vi "Compute Pseudo-Phase Lifetime Plot.vi"(8 "Error In":errorcluster, 9 "Compute Delta Tau":bool, 10 "Phasor Parameters":T1={"Display Parameters"={"# Points"=0, "Ramp Type"=enum."Linear", "Type of Series"=enum."1-Exp Decays", "Min tau"=0.0, "Max tau"=0.0, "Include 0"=FALSE, "Include Infinity"=FALSE}, "Phasor Parameters"={"Harmonic frequency"=0.0, "Use f* = 1/D Frequency"=FALSE, "Calibrated Phasor"=FALSE, "Calibration Lifetime"=1e-09, "Phasor Calculation"=enum."Direct Sum", "SEPL Type"=enum."UC", "# Gates"=1.0, "Square Gate Width"=1e-09, "Show Ticks"=FALSE}, "Decay & IRF Parameters"={"Lifetime"=0.0, "IRF Offset"=0.0, "Laser Period"=0.0, "Normalized Decays"=FALSE, "IRF Model"=enum."Dirac", "IRF Parameter 1"=0.0}, "Gate Parameters"={"First Gate Start"=0.0, "Use Gate Center"=FALSE, "Gate Width"=0.0, "Gate Step"=0.0, "# Gates"=0.0, "Gate Type"=enum."Square", "Edge Width"=0.0, "Top Slope"=0.0, "Reversed Sawtooth?"=FALSE, "Analytical Computation"=FALSE, "Tolerance"=1.0, "Integration"=enum."Item 0", "# Steps"=1.0, "Type of User-defined Function"=enum."Gate"}, "Detector Parameters"={"Frames/Image"=0, "Gates/Frame"=0, "Bits/Frame"=0, "Multiplicity"=0, "Incident Signal"=0.0}} {"Detector Parameters"."Frames/Image" min=1; "Detector Parameters"."Multiplicity" min=0; "Detector Parameters"."Bits/Frame" min=1; "Detector Parameters"."Gates/Frame" min=1; "Gate Parameters"."# Steps" min=0.0; "Gate Parameters"."Tolerance" min=0.0; "Gate Parameters"."Top Slope" min=0.0; "Gate Parameters"."Edge Width" min=0.0; "Gate Parameters"."Gate Step" min=0.0; "Gate Parameters"."# Gates" min=0.0 step=1.0; "Gate Parameters"."Gate Width" min=0.0; "Decay & IRF Parameters"."Lifetime" min=0.0; "Decay & IRF Parameters"."Laser Period" min=0.0; "Phasor Parameters"."Square Gate Width" min=0.0; "Phasor Parameters"."# Gates" min=0.0; "Phasor Parameters"."Calibration Lifetime" min=0.0; "Phasor Parameters"."Harmonic frequency" min=0.0; "Display Parameters"."Min tau" min=0.0; "Display Parameters"."Max tau" min=0.0; "Display Parameters"."# Points" min=1 step=1}, 11 "P-tau_ph(tau) Graph Refnum":refnum<vi>) -> (0 "Error Out":errorcluster)   [LabVIEW 2019]
uses:
  Pseudo Phasor Parameters.ctl
  Phasor Explorer Display Parameters.ctl
  Type of Series.ctl
  Phasor Explorer Phasor Parameters.ctl
  Phasor Calculation Type.ctl
  Phasor Type.ctl
  Phasor Explorer Decay Parameters.ctl
  IRF Model.ctl
  Phasor Explorer Gate Parameters.ctl
  Gate Type.ctl
  Phasor Explorer Detector Parameters.ctl
  Phasor UC_N[W] Parameters.ctl
  <vilib>/Utility/error.llb/Error Cluster From Error Code.vi
  SEPXP Globals.vi
  <vilib>/ErrorRing/Error Ring.xnode
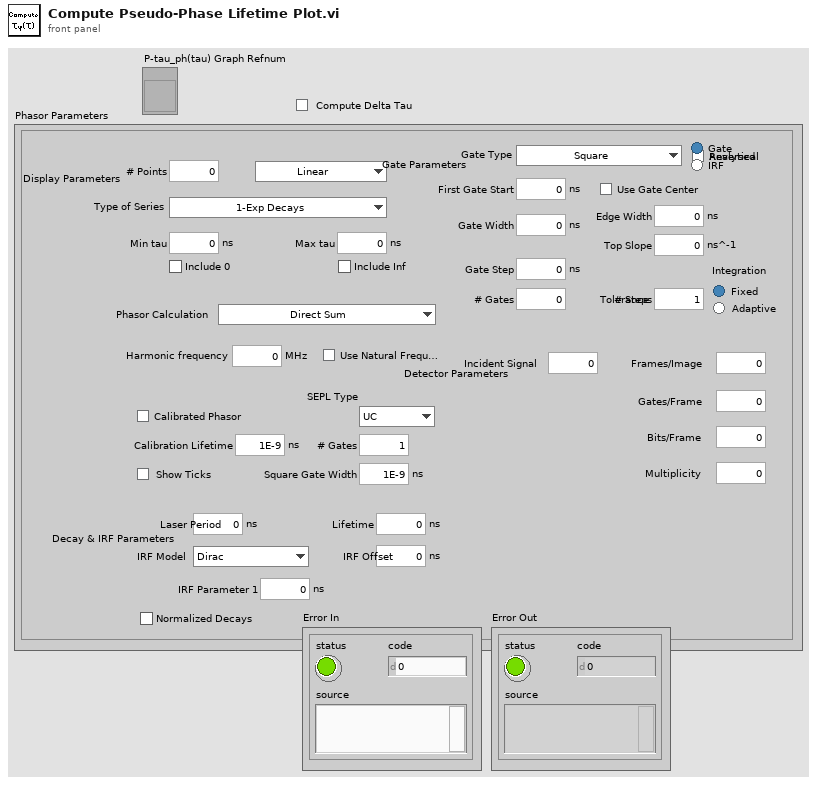
[diagram p1: front panel]
types:
  T1 = typedef "Pseudo Phasor Parameters.ctl" = cluster{"Display Parameters":T2, "Phasor Parameters":T4, "Decay & IRF Parameters":T7, "Gate Parameters":T9, "Detector Parameters":T11}
  T2 = typedef "Phasor Explorer Display Parameters.ctl" = cluster{"# Points":i32, "Ramp Type":enum16{"Linear", "Logarithmic"}, "Type of Series":T3, "Min tau":dbl[unit], "Max tau":dbl[unit], "Include 0":bool, "Include Infinity":bool}
  T3 = typedef "Type of Series.ctl" = enum16{"1-Exp Decays", "Linear Combination of 1-Exp"}
  T4 = typedef "Phasor Explorer Phasor Parameters.ctl" = cluster{"Harmonic frequency":dbl[unit], "Use f* = 1/D Frequency":bool, "Calibrated Phasor":bool, "Calibration Lifetime":dbl[unit], "Phasor Calculation":T5, "SEPL Type":T6, "# Gates":dbl, "Square Gate Width":dbl[unit], "Show Ticks":bool}
  T5 = typedef "Phasor Calculation Type.ctl" = enum16{"Direct Sum", "Analytical Formula"}
  T6 = typedef "Phasor Type.ctl" = enum16{"UC", "L_N", "L_N[W]"}
  T7 = typedef "Phasor Explorer Decay Parameters.ctl" = cluster{"Lifetime":dbl[unit], "IRF Offset":dbl[unit], "Laser Period":dbl[unit], "Normalized Decays":bool, "IRF Model":T8, "IRF Parameter 1":dbl[unit]}
  T8 = typedef "IRF Model.ctl" = enum16{"Dirac", "Exponential"}
  T9 = typedef "Phasor Explorer Gate Parameters.ctl" = cluster{"First Gate Start":dbl[unit], "Use Gate Center":bool, "Gate Width":dbl[unit], "Gate Step":dbl[unit], "# Gates":dbl, "Gate Type":T10, "Edge Width":dbl[unit], "Top Slope":dbl[unit], "Reversed Sawtooth?":bool, "Analytical Computation":bool, "Tolerance":dbl, "Integration":enum32{"Item 0", "Item 1"}, "# Steps":dbl, "Type of User-defined Function":enum32{"Gate", "IRF"}}
  T10 = typedef "Gate Type.ctl" = enum16{"Square", "Finite Edge Square", "Finite Edge, Tilted Top Square", "Triangle", "Sawtooth", "User-defined"}
  T11 = typedef "Phasor Explorer Detector Parameters.ctl" = cluster{"Frames/Image":i32, "Gates/Frame":i32, "Bits/Frame":i32, "Multiplicity":i32, "Incident Signal":dbl}
  T12 = typedef "Phasor UC_N[W] Parameters.ctl" = cluster{"Laser Period":dbl[unit], "Gate Width":dbl[unit], "Gate Step":dbl[unit], "Harmonic frequency":dbl[unit], "IRF offset":dbl[unit], "# Gates":dbl}
  T13 = typedef "Gate Definitions.ctl" = cluster{"First Gate: t1":ext, "Gate Width: W":ext, "Gate Step: d":ext, "# Gates: G":ext, "Use Gate Center":bool, "Frames/Image: F":i32, "Gates/Frame: L":i32, "Bits/Frame: q":i32, "Multiplicity: p":i32, "Gate Type":T10, "Gate Edge s":ext, "Gate Top Slope":ext, "Reversed Sawtooth?":bool, "Computation":bool, "User-defined Gate":T14, "Tolerance":ext, "Integration":enum32{"Item 0", "Item 1"}, "# Steps":ext, "Type of User-defined Function":enum32{"Gate", "IRF"}}
  T14 = typedef "XY Plot Data.ctl" = cluster{"X Array":dbl[], "Y Array":dbl[]}
  T15 = typedef "Decay Definiton.ctl" = cluster{"offset: t0":ext, "period: T":ext, "lifetime: tau":ext, "Incident Signal: I":ext, "Normalized Decays":bool, "IRF Model":T8, "IRF Parameter 1":ext}
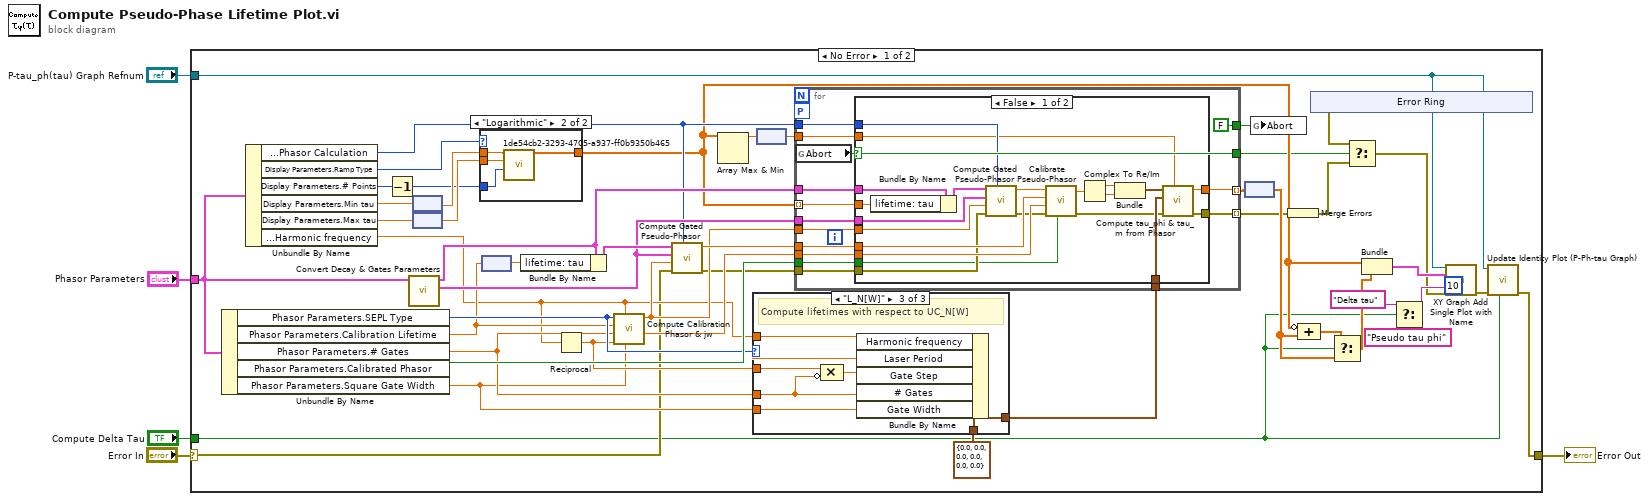
[diagram p0: block diagram]
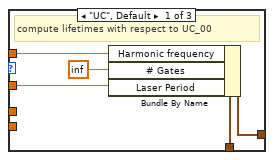
[diagram p2: hidden frame]
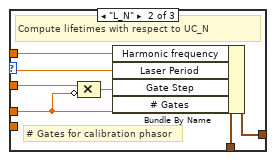
[diagram p3: hidden frame]
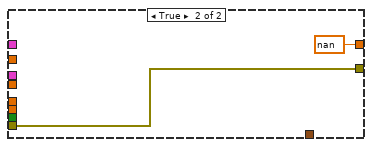
[diagram p4: hidden frame]
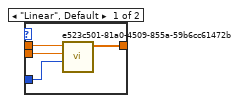
[diagram p5: hidden frame]
diagram:
  n1 = case shown="No Error" "Error In" {
    selector: "Error In" -> [w8 w122]
    tunnel: "Phasor Parameters" -> [w22 _]
    tunnel: "P-tau_ph(tau) Graph Refnum" -> [w41 _]
    tunnel: [w39 w122] -> w2
    tunnel: "Compute Delta Tau" -> [w6 _]
    frame No Error {
      (unwired) 10 ("Max Legend Size (8)")
      n2 = Unbundle By Name(w22) -> ("Phasor Parameters.SEPL Type"=w23:T6, "Phasor Parameters.Calibration Lifetime"=w18:dbl[unit], "Phasor Parameters.# Gates"=w19:dbl, "Phasor Parameters.Calibrated Phasor"=w36:bool, "Phasor Parameters.Square Gate Width"=w11:dbl[unit])
      n3 = Unbundle By Name(w22) -> ("Phasor Parameters.Phasor Calculation"=w35:T5, "Display Parameters.Ramp Type"=w44:enum16{"Linear", "Logarithmic"}, "Display Parameters.# Points"=w43:i32, "Display Parameters.Min tau"=w52:dbl[unit], "Display Parameters.Max tau"=w53:dbl[unit], "Phasor Parameters.Harmonic frequency"=w17:dbl[unit])
      n4 = Decrement(x=w43) -> (x-1=w42:i32)
      n5 = call "Convert Decay & Gates Parameters.vi"("Phasor Parameters"=w22) -> ("Gates Definitions"=w37:T13, "Decay Definition"=w38:T15)  [unwired: 9 in]
      n6 = node(w52) -> (w46:dbl)
      n7 = node(w53) -> (w47:dbl)
      n8 = case shown="\"Logarithmic\"" w44 {
        tunnel: w47 -> [w117 w119]
        tunnel: w46 -> [w116 w120]
        tunnel: [w115 w118] -> w26
        tunnel: w42 -> [w114 w121]
        frame "Linear", Default {
          n9 = call "e523c501-81a0-4509-855a-59b6cc61472b.vi"("# Steps (1)"=w114, "End (1)"=w117, "Start (0)"=w116) -> ("Ramp"=w115:dbl[])  [unwired: 7 in, 1 out]
        }
        frame "Logarithmic" {
          n10 = call "1de54cb2-3293-4705-a937-ff0b9350b465.vi"("# Steps (1)"=w121, "End (1)"=w119, "Start (1)"=w120) -> ("Ramp"=w118:dbl[])  [unwired: 7 in, 1 out]
        }
      }
      n11 = node(w18) -> (w49:dbl)
      n12 = Bundle By Name(cluster=w38, "lifetime: tau"=w49) -> (w50:T15)
      n13 = Reciprocal(x=w17) -> (1/x=w16:dbl[unit])
      n14 = call "Compute Calibration Phasor & jw.vi"("Gate Width"=w11, "Harmonic frequency"=w17, "Laser Period"=w16, "# Gates"=w19, "Calibration Lifetime"=w18, "Calibration Phasor Type"=w23) -> ("z (tau_cal)"=w27:cdb, "i 2 pi f (GHz)"=w28:cdb)  [unwired: 4 in]
      n15 = call "Compute Gated Pseudo-Phasor.vi"("Phasor Calculation Type"=w35, "Error In"=w8, "j 2 pi f"=w28, "Gates Definitions"=w37, "Decay Definition"=w50) -> ("Error Out"=w10:errorcluster, "phasor"=w48:cxt)  [unwired: 4 in, 1 out]
      n16 = Array Max & Min(array=w26) -> (max value=w25:dbl)  [unwired: 3 out]
      n17 = case shown="\"L_N[W]\"" w23 {
        tunnel: [w62 w68 w75] -> w21
        tunnel: T12 {"Laser Period"=0.0, "Gate Width"=0.0, "Gate Step"=0.0, "Harmonic frequency"=0.0, "IRF offset"=0.0, "# Gates"=0.0} ("Phasor UCN[W] Parameters") -> [w60 w67 w74]
        tunnel: w16 -> [w59 w64 w71]
        tunnel: w17 -> [w58 w66 w73]
        tunnel: w19 -> [_ w65 w72]
        tunnel: w11 -> [_ _ w69]
        frame "UC", Default {
          # "compute lifetimes with respect to UC_00"
          n18 = Bundle By Name(cluster=w60, "Harmonic frequency"=w58, "# Gates"=inf ("Gate Parameters.# Gates"), "Laser Period"=w59) -> (w62:T12)
        }
        frame "L_N" {
          # "# Gates for calibration phasor"
          # "Compute lifetimes with respect to UC_N"
          n19 = Compound Arithmetic op=MULTIPLY(w64, invert w65) -> (w63:dbl[unit])
          n20 = Bundle By Name(cluster=w67, "Harmonic frequency"=w66, "Laser Period"=w64, "Gate Step"=w63, "# Gates"=w65) -> (w68:T12)
        }
        frame "L_N[W]" {
          # "Compute lifetimes with respect to UC_N[W]"
          n21 = Compound Arithmetic op=MULTIPLY(w71, invert w72) -> (w70:dbl[unit])
          n22 = Bundle By Name(cluster=w74, "Harmonic frequency"=w73, "Laser Period"=w71, "Gate Step"=w70, "# Gates"=w72, "Gate Width"=w69) -> (w75:T12)
        }
      }
      n23 = node(w25) -> (w24:dbl[unit])
      n24 = for {
        tunnel: w48 -> [w90]
        tunnel: w27 -> [w89]
        tunnel: w36 -> [w88]
        tunnel: w28 -> [w87]
        tunnel: w37 -> [w84]
        tunnel: w38 -> [w85]
        tunnel: w26 -> [w86] mode=indexing
        tunnel: [w81] -> w45 mode=indexing
        tunnel: w35 -> [w83]
        tunnel: w24 -> [w82]
        tunnel: w21 -> [w80]
        workers-P: _ -> [_]
        tunnel: [FALSE ("Abort")] -> w15
        tunnel: [w78] -> w14
        tunnel: [w77] -> w9 mode=indexing
        tunnel: w10 -> [w76]
        n25 = global read "SEPXP Globals.vi" "Abort"() -> (w78:bool)
        n26 = case shown="False" w78 {
          tunnel: w90 -> [w111 _]
          tunnel: w89 -> [w110 _]
          tunnel: w88 -> [w93 _]
          tunnel: w87 -> [w109 _]
          tunnel: w86 -> [w108 _]
          tunnel: w85 -> [w107 _]
          tunnel: w84 -> [w105 _]
          tunnel: w83 -> [w100 _]
          tunnel: w82 -> [w97 _]
          tunnel: [w98 dbl[unit] nan ("tau_ph")] -> w81
          tunnel: w80 -> [w96 _]
          tunnel: [w95 w112] -> w77
          tunnel: w76 -> [w94 w112]
          frame False {
            n27 = Bundle By Name(cluster=w107, "lifetime: tau"=w108) -> (w106:T15)
            n28 = call "Compute Gated Pseudo-Phasor.vi"("Phasor Calculation Type"=w100, "Error In"=w94, "j 2 pi f"=w109, "Gates Definitions"=w105, "Decay Definition"=w106) -> ("Error Out"=w92:errorcluster, "phasor"=w104:cxt)  [unwired: 4 in, 1 out]
            n29 = call "Calibrate Pseudo-Phasor.vi"("Calibrated Phasor"=w93, "Error In"=w92, "Target Phasor"=w110, "Calibration Pseudo-Phasor"=w111, "Pseudo-Phasor in"=w104) -> ("Error Out"=w91:errorcluster, "Pseudo-Phasor out"=w103:cxt)  [unwired: 5 in]
            n30 = Complex To Re/Im(x + iy=w103) -> (x=w102:ext, y=w101:ext)
            n31 = Bundle(w102, w101) -> (w99:cluster{ext, ext})  [unwired: 1 in]
            n32 = call "Compute tau_phi & tau_m from Phasor.vi"("max tau"=w97, "Error In"=w91, "Phasor UCN[W] Parameters"=w96, "Phasor"=w99) -> ("Error Out"=w95:errorcluster, "tau_ph"=w98:dbl[unit])  [unwired: 5 in, 1 out]
          }
          frame True {
          }
        }
      }
      n33 = node(w45) -> (w33:dbl[])
      n34 = global write "SEPXP Globals.vi" "Abort"(w15) -> ()
      n35 = Merge Errors(w9) -> (w7:errorcluster)
      n36 = Compound Arithmetic op=ADD(invert w26, w33) -> (w32:dbl[])
      n37 = xnode "Error Ring"() -> ("error out"=w13:errorcluster)
      n38 = Select(t=w32, s=w6, f=w33) -> (s? t:f=w34:dbl[])
      n39 = Select(t=w13, s=w14, f=w7) -> (s? t:f=w12:errorcluster)
      n40 = Bundle("Ramp"=w26, w34) -> (w51:cluster{"Ramp":dbl[], dbl[]})  [unwired: 1 in]
      n41 = Select(t="Delta tau" ("Plot Name (\"Plot\")"), s=w6, f="Pseudo tau phi" ("Plot Name (\"Plot\")")) -> (s? t:f=w31:string)
      n42 = call "XY Graph Add Single Plot with Name.vi"("XYGraph Ref in"=w41, "Plot"=w51, "Plot Name (\"Plot\")"=w31, "error in (no error)"=w12) -> ("error out"=w40:errorcluster)  [unwired: 8 in, 3 out]
      n43 = call "Update Identity Plot (P-Ph-tau Graph).vi"("Delta tau"=w6, "error in (no error)"=w40, "XYGraph in"=w41) -> ("error out"=w39:errorcluster)  [unwired: 8 in]
    }
    frame Error {
    }
  }
  "Error Out" <- w2
